vi "AWGSendPulseArrayContinuous.vi"(8 "error in (no error)":errorcluster, 10 "Step Number":i32, 11 "AWG pulses array":variant[](array[variant])) -> (0 "error out":errorcluster, 3 "msg out":string)   [LabVIEW 2019]
panel:
  in  "Sample rate":dbl=500000000.0 format="%^#_6g"
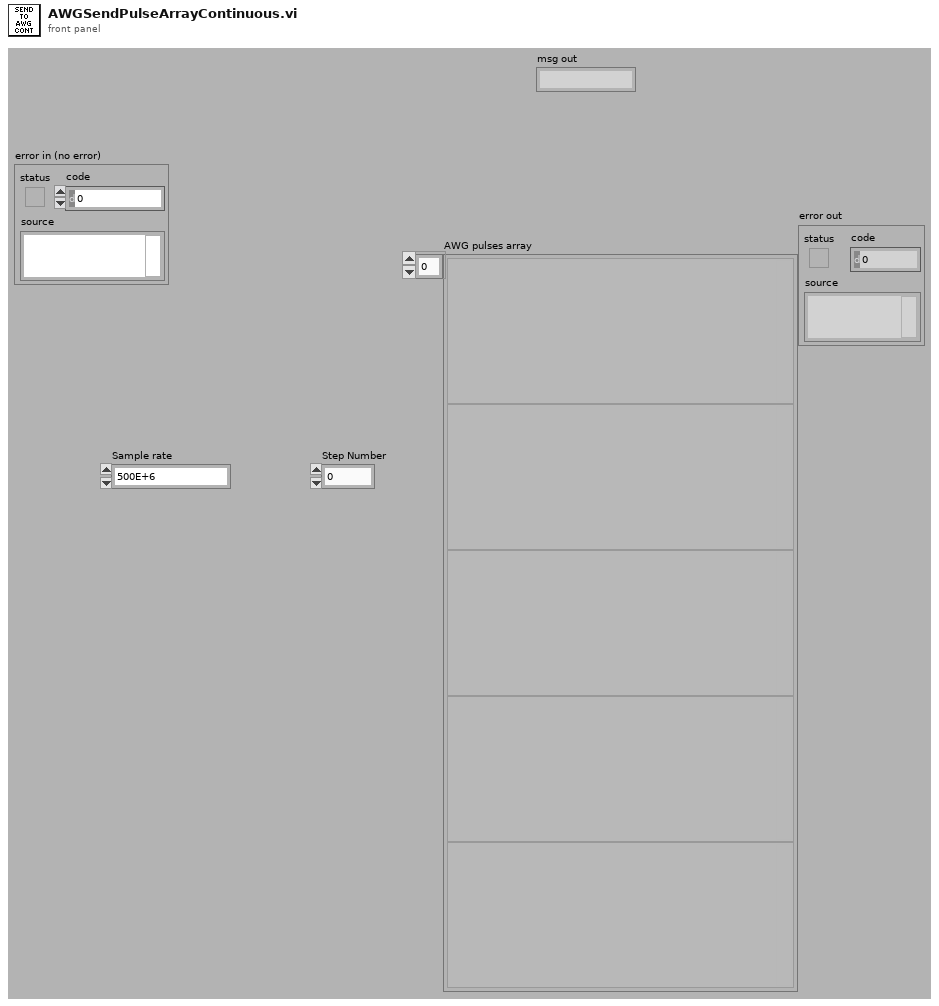
[diagram p1: front panel]
types:
  T1 = cluster{"Sample rate":dbl, "Step Number":i32, "Array":variant[], "mVpp":dbl}
  T2 = cluster{"Sample rate":dbl, "Step Number":i32, "AWG pulses array":variant[], dbl}
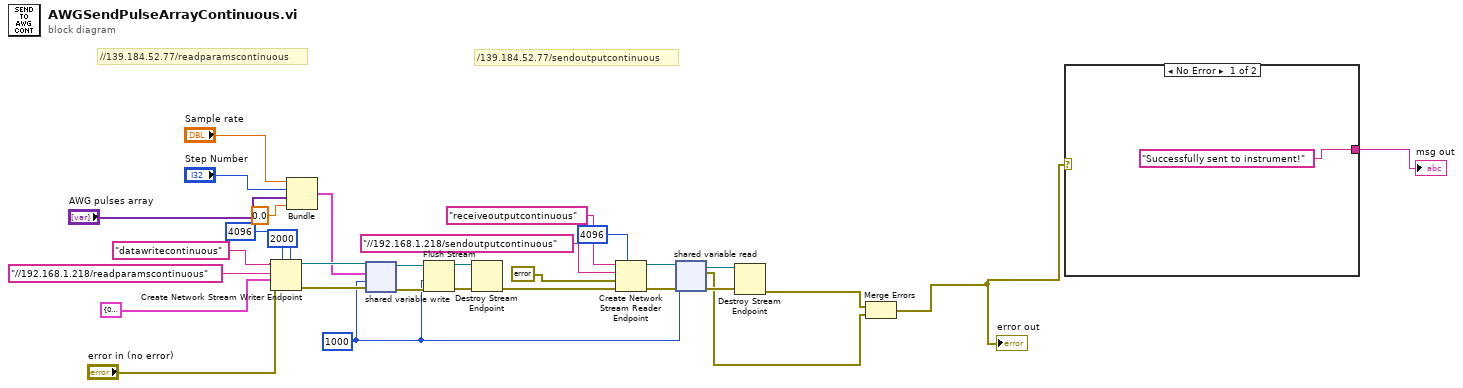
[diagram p0: block diagram]
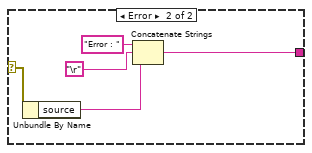
[diagram p2: hidden frame]
diagram:
  w3 = 1000 ("timeout ms (-1)")
  # "/139.184.52.77/sendoutputcontinuous"
  # "//139.184.52.77/readparamscontinuous"
  n1 = Create Network Stream Writer Endpoint(5:2000 ("timeout in ms (-1)"), 7:4096 ("writer buffer size"), 8:"error in (no error)", 9:T1 {"Sample rate"=0.0, "Step Number"=0, "Array"=[], "mVpp"=0.0} ("output cluster"), 10:"//192.168.1.218/readparamscontinuous" ("reader url"), 11:"datawritecontinuous" ("writer name")) -> (0:w21:errorcluster, 3:w22:refnum<k21>)  [unwired: 1 in]
  n2 = Bundle("Sample rate"="Sample rate", "Step Number"="Step Number", "AWG pulses array"="AWG pulses array", 0.0) -> (w14:T2)  [unwired: 1 in]
  n3 = shared-variable-write(w22, w21, w14, w3) -> (w20:refnum<k21>, w19:errorcluster)  [unwired: 1 out]
  n4 = Flush Stream(8:w19, 9:w3, 11:w20) -> (0:w31:errorcluster, 3:w30:refnum<k21>)  [unwired: 1 in, 1 out]
  n5 = Destroy Stream Endpoint(8:w31, 11:w30) -> (0:w11:errorcluster)
  n6 = Create Network Stream Reader Endpoint(7:4096 ("reader buffer size"), 8:w11, 9:errorcluster {"status"=FALSE, "code"=0, "source"=""} ("error out"), 10:"//192.168.1.218/sendoutputcontinuous" ("writer url"), 11:"receiveoutputcontinuous" ("reader name")) -> (0:w27:errorcluster, 3:w28:refnum<k21>)  [unwired: 2 in]
  n7 = shared-variable-read(w28, w27, w3) -> (w26:refnum<k21>, w25:errorcluster, w7:errorcluster)  [unwired: 1 out]
  n8 = Destroy Stream Endpoint(8:w25, 11:w26) -> (0:w10:errorcluster)
  n9 = Merge Errors(w10, w7) -> (w1:errorcluster)
  "error out" <- w1
  n10 = case shown="No Error" w1 {
    selector: w1 -> [_ w35]
    tunnel: ["Successfully sent to instrument!" w33] -> w4
    frame No Error {
    }
    frame Error {
      n11 = Unbundle By Name(w35) -> ("source"=w34:string)
      n12 = Concatenate Strings("Error : " ("string"), "\r", w34) -> (w33:string)
    }
  }
  "msg out" <- w4
